vi "GetAllInfo.vi"(8 "Error in":errorcluster, 11 "base path":path) -> (0 "Error out":errorcluster, 3 "Account Info":T1)   [LabVIEW 2017]
doc: "This VI initially read all the account info and stores it in temporary memory for the future access"
uses:
  <vilib>/Utility/file.llb/Read From Spreadsheet File (string).vi
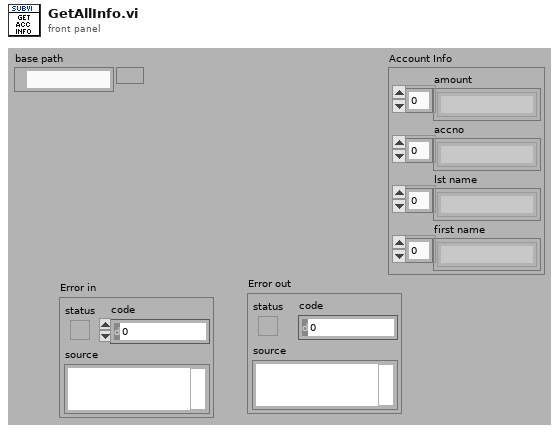
[diagram p1: front panel]
types:
  T1 = cluster{"amount":string[], "accno":string[], "lst name":string[], "first name":string[]}
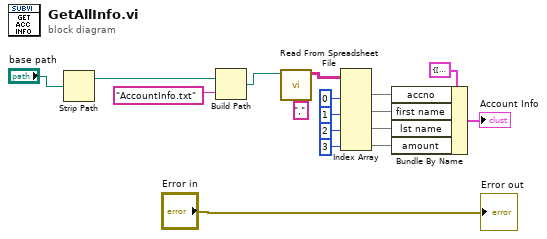
[diagram p0: block diagram]
diagram:
  n1 = Strip Path(path="base path") -> (stripped path=w1:path)  [unwired: 1 out]
  n2 = Build Path(base path=w1, name or relative path="AccountInfo.txt") -> (appended path=w17:path)
  n3 = call-poly <vilib>:"Read From Spreadsheet File.vi"("delimiter (\\t)"="," ("delimiter (\\t)"), "file path (dialog if empty)"=w17) -> ("all rows"=w15:string[][])  [unwired: 5 in, 4 out]
  n4 = Index Array(array=w15, index (col) #1=0 ("disabled index (col)"), index (col) #2=1 ("index (col)"), index (col) #3=2 ("index (col)"), index (col) #4=3 ("index (col)")) -> (element #1=w13:string[], element #2=w12:string[], element #3=w11:string[], element #4=w10:string[])  [unwired: 4 in]
  n5 = Bundle By Name(cluster=T1 {"amount"=[], "accno"=[], "lst name"=[], "first name"=[]}, "accno"=w13, "first name"=w12, "lst name"=w11, "amount"=w10) -> (→"Account Info":T1)
  "Error out" <- "Error in"
